vi "Query Multi Eval Meas List ES Flatness Ripple Limit Check Results.vi"(7 "Result Type (Current)":i32(ring) items=["Current", "Average", "Extreme"], 8 "error in (no error)":errorcluster, 9 "Ripple (Ripple 1)":T1=1 items=["Ripple 1"=1, "Ripple 2"=2], 10 "Instance (1)":T2=1, 11 "VISA resource name":refnum<visa-resource-name>) -> (0 "error out":errorcluster, 1 "ES Flatness RIpple Limit Check Results":i32[](array[numeric]), 2 "Reliability":i32, 3 "VISA resource name out":refnum<visa-resource-name>)   [LabVIEW 2020, in "Rohde&Schwarz CMXP NR FR2 Measurement.lvlib"]
doc: "Returns the limit check results for equalizer spectrum flatness single value results (ripple 1 or ripple 2) for all measured list mode segments.\n\nAttributes:\nRSCMXPNRFR2M_ATTR_QUERY_MULTI_EVAL_MEASUREMENT_LIST_ESF_RIPPLE_AVERAGE_LIMIT_CHECK_RESULTS\nRSCMXPNRFR2M_ATTR_QUERY_MULTI_EVAL_MEASUREMENT_LIST_ESF_RIPPLE_CURRENT_LIMIT_CHECK_RESULTS\nRSCMXPNRFR2M_ATTR_QUERY_MULTI_EVAL_MEASUREMENT_LIST_ESF_RIPPLE_EXTREME_LIMIT_CHECK_RESULTS\n\nRemote-control commands:\nCALCulate:NRMMw:MEAS<i>:MEValuation:LIST:ESFLatness:RIPPle<no>:AVERage?\nCALCulate:NRMMw:MEAS<i>:MEValuation:LIST:ESFLatness:RIPPle<no>:CURRent?\nCALCulate:NRMMw:MEAS<i>:MEValuation:LIST:ESFLatness:RIPPle<no>:EXTReme?"
uses:
  <instrlib>/Rohde&Schwarz CMXP NR FR2 Measurement/Rohde&Schwarz CMXP NR FR2 Measurement.lvlib
  <instrlib>/Rohde&Schwarz CMXP NR FR2 Measurement/Private/_Instance.ctl
  <instrlib>/Rohde&Schwarz CMXP NR FR2 Measurement/Private/_Ripple.ctl
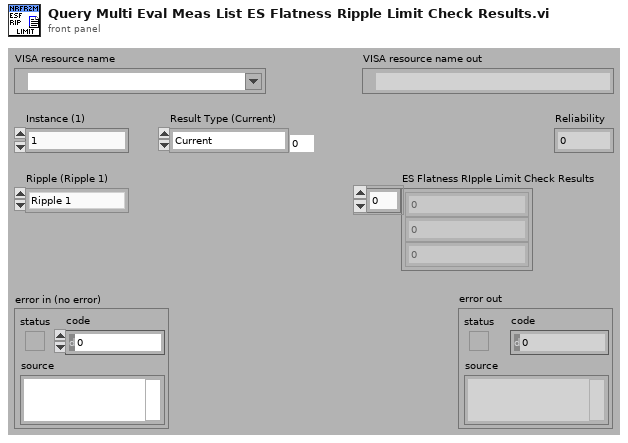
[diagram p1: front panel]
types:
  T1 = typedef "Rohde&Schwarz CMXP NR FR2 Measurement.lvlib/_Ripple.ctl" = i32
  T2 = typedef "Rohde&Schwarz CMXP NR FR2 Measurement.lvlib/_Instance.ctl" = i32
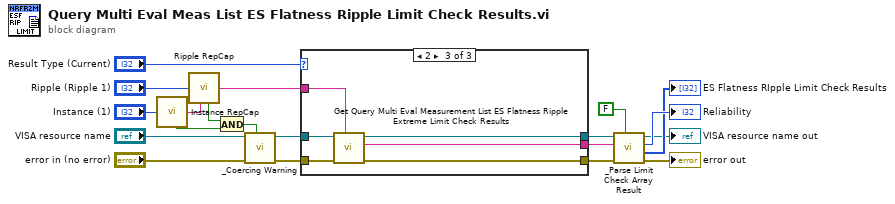
[diagram p0: block diagram]
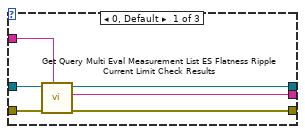
[diagram p2: hidden frame]
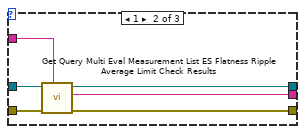
[diagram p3: hidden frame]
diagram:
  n1 = call <instrlib>:"Instance RepCap.vi"("Instance In"="Instance (1)") -> ("In Range?"=w18:bool, "RepCap Identifier Out"=w1:string)  [unwired: 1 in]
  n2 = call <instrlib>:"Ripple RepCap.vi"("Ripple In"="Ripple (Ripple 1)", "RepCap String In (\"\")"=w1) -> ("In Range?"=w20:bool, "RepCap Identifier Out"=w12:string)
  n3 = And(x=w20, y=w18) -> (x .and. y?=w19:bool)
  n4 = call <instrlib>:"_Coercing Warning.vi"("In Range?"=w19, "error in (no error)"="error in (no error)", "VISA resource name"="VISA resource name") -> ("error out"=w14:errorcluster, "VISA resource name out"=w13:refnum<visa-resource-name>)  [unwired: 7 in]
  n5 = case shown="2" "Result Type (Current)" {
    tunnel: w14 -> [w26 w32 w38]
    tunnel: w13 -> [w25 w31 w37]
    tunnel: w12 -> [w24 w30 w36]
    tunnel: [w23 w29 w35] -> w10
    tunnel: [w22 w28 w34] -> w9
    tunnel: [w21 w27 w33] -> w8
    frame 0, Default {
      n6 = call "Get Query Multi Eval Measurement List ES Flatness Ripple Current Limit Check Results"("Repeated Capabilities"=w24, "error in (no error)"=w26, "instrument handle"=w25) -> ("error out"=w23:errorcluster, "Query Multi Eval Measurement List ES Flatness Ripple Current Limit Check Results"=w22:string, "instrument handle out"=w21:refnum<visa-resource-name>)  [unwired: 6 in]
    }
    frame 1 {
      n7 = call "Get Query Multi Eval Measurement List ES Flatness Ripple Average Limit Check Results"("Repeated Capabilities"=w30, "error in (no error)"=w32, "instrument handle"=w31) -> ("error out"=w29:errorcluster, "Query Multi Eval Measurement List ES Flatness Ripple Average Limit Check Results"=w28:string, "instrument handle out"=w27:refnum<visa-resource-name>)  [unwired: 6 in]
    }
    frame 2 {
      n8 = call "Get Query Multi Eval Measurement List ES Flatness Ripple Extreme Limit Check Results"("Repeated Capabilities"=w36, "error in (no error)"=w38, "instrument handle"=w37) -> ("error out"=w35:errorcluster, "Query Multi Eval Measurement List ES Flatness Ripple Extreme Limit Check Results"=w34:string, "instrument handle out"=w33:refnum<visa-resource-name>)  [unwired: 6 in]
    }
  }
  n9 = call <instrlib>:"_Parse Limit Check Array Result.vi"("error in (no error)"=w10, "Input String"=w9, "VISA resource name"=w8, "Out of tolerance? (F)"=FALSE) -> ("error out"=→"error out":errorcluster, "Results"=→"ES Flatness RIpple Limit Check Results":i32[], "Reliability"=→"Reliability":i32, "VISA resource name out"=→"VISA resource name out":refnum<visa-resource-name>)  [unwired: 3 in]
